vi "read_data_linear_z_single(SubVI).vi"(8 "error in (no error)":errorcluster) -> (0 "error out":errorcluster, 3 "number":dbl[](array[numeric]))   [LabVIEW 2014]
uses:
  <vilib>/xml/Load XML String.vi
  <vilib>/xml/Close Reference(Node).vi
  Program Files (x86)/National Instruments/LabVIEW 2014/vi.lib/addons/internet/NI_InternetTK_Core_VIs.lvlib
  <vilib>/xml/NI_XML.lvlib
  <resource>/objmgr/DOMUserDefRef.rc
panel:
  out "content":string
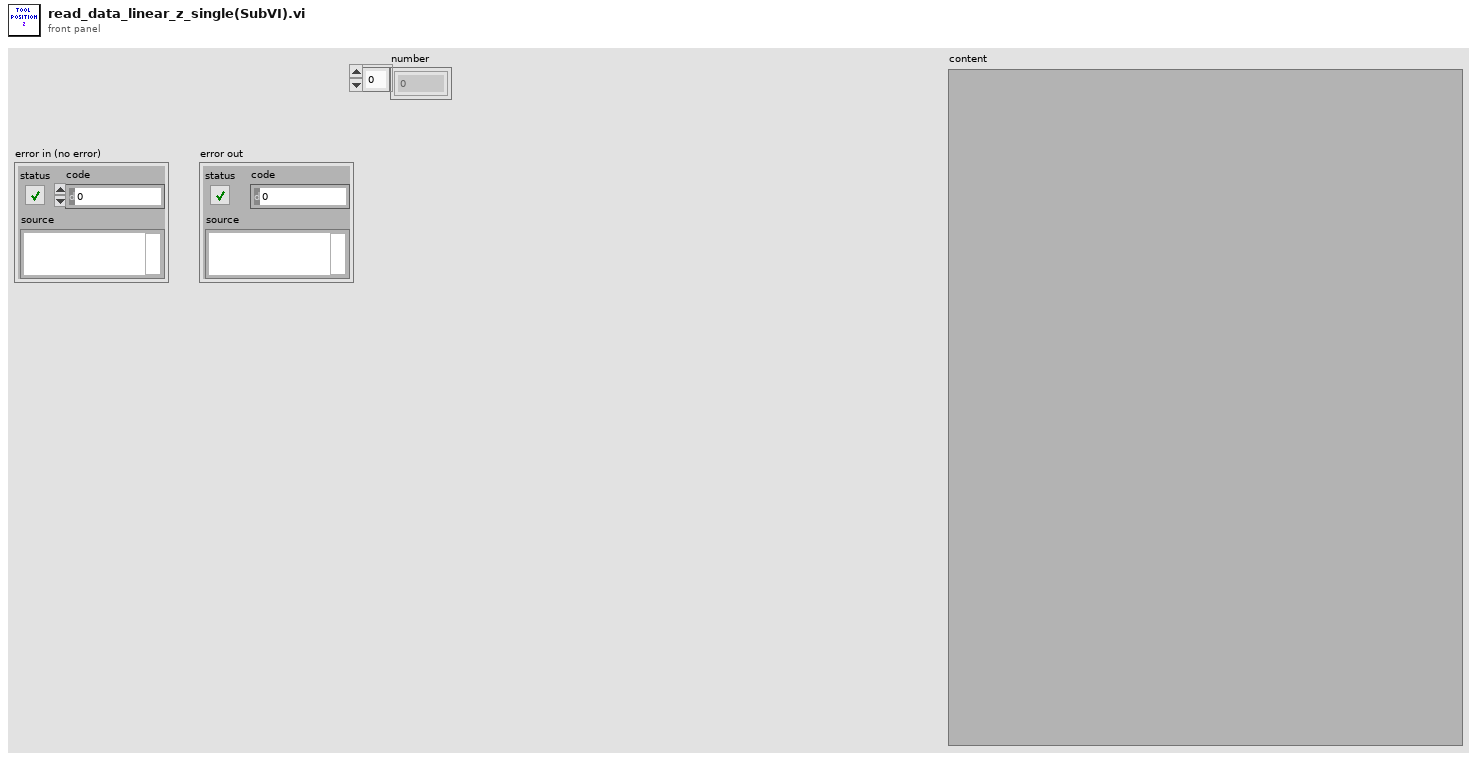
[diagram p1: front panel]
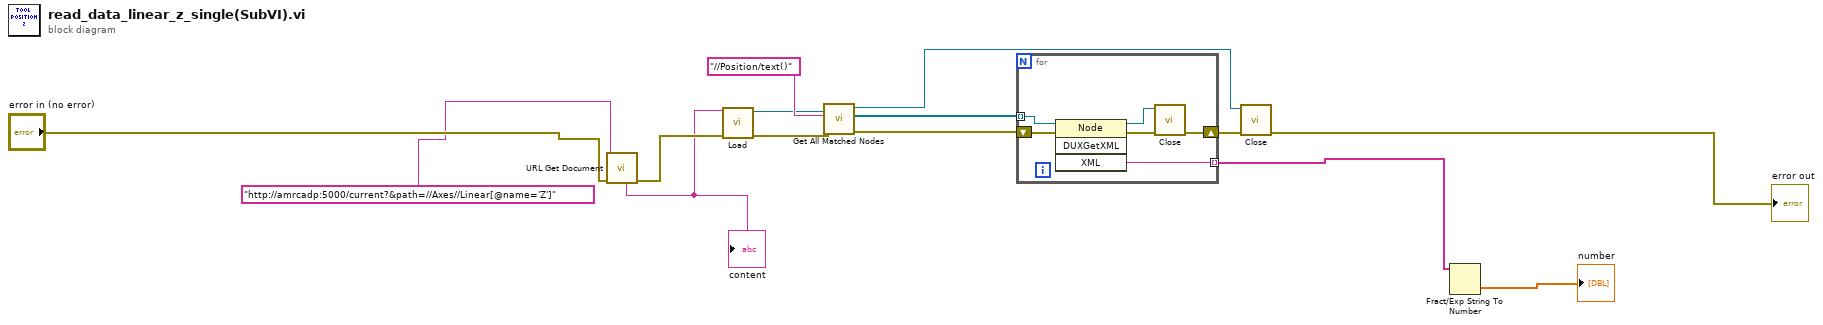
[diagram p0: block diagram]
diagram:
  n1 = call "URL Get Document.vi"("error in (no error)"="error in (no error)", "URL"="http://amrcadp:5000/current?&path=//Axes//Linear[@name='Z']") -> ("error out"=w12:errorcluster, "content"=w9:string)  [unwired: 5 in, 3 out]
  "content" <- w9
  n2 = call-poly <vilib>:"Load.vi"("XML string"=w9, "error in (no error)"=w12) -> ("DOM document out"=w6:refnum<k20>, "error out"=w7:errorcluster)  [unwired: 11 in, 1 out]
  n3 = call <vilib>:"Get All Matched Nodes.vi"("error in (no error)"=w7, "XPath expression"="//Position/text()", "node in"=w6) -> ("error out"=w4:errorcluster, "node result array"=w3:refnum<k20>[], "node out"=w8:refnum<k20>)  [unwired: 6 out]
  n4 = for {
    tunnel: w3 -> [w16] mode=indexing
    shift-right: [w18] -> w5
    shift-left: w4 -> [w17]
    tunnel: [w15] -> w2 mode=indexing
    n5 = invoke on="Invoke Node" class="Node" method="DUXGetXML"(reference=w16, error in=w17) -> (reference out=w19:refnum<k20>, error out=w20:errorcluster, "XML"=w15:string)  [unwired: 2 in, 1 out]
    n6 = call-poly <vilib>:"Close.vi"("error in (no error)"=w20, "node"=w19) -> ("error out"=w18:errorcluster)  [unwired: 7 out]
  }
  n7 = call-poly <vilib>:"Close.vi"("error in (no error)"=w5, "node"=w8) -> ("error out"=→"error out":errorcluster)  [unwired: 7 out]
  n8 = Fract/Exp String To Number(string=w2) -> (number=→"number":dbl[])  [unwired: 3 in, 1 out]
